vi "WiFiCheck.vi"() -> ()   [LabVIEW 2016]
uses:
  VIs/uPythonX/uPythonX.xctl
panel:
  in  "All Combined":T1(xcontrol)={"VISA Refnum in"="ASRL30::INSTR", "Python Code"="import machine, network, ubinascii, ujson, urequests\nfrom pyb import DAC\nimport utime,math\n\nimport stm\nQSPI = 0xa0001000\nstm.mem32[QSPI] = 0x5000319\nstm.mem32[QSPI+4] = 0x140700\n\nWiFi = network.WLAN()\ndac = DAC(1,buffering=True)            # create DAC 1 on pin X5\n\ndef connect():\n     EN1 = machine.Pin(\"W23\", machine.Pin.OUT, value=1)  # set power high for USB power (500mA now allowed)\n     if not WiFi.isconnected():\n          print (\"Connecting ..\")\n          WiFi.active(True)\n          WiFi.connect(\"Tufts_Wireless\",\"\")\n          i=0\n          while i < 25 and not WiFi.isconnected():\n               utime.sleep_ms(200)\n               i=i+1\n          if WiFi.isconnected():\n               print (\"Connection succeeded\")\n          else:\n               print (\"Connection failed\")     \n\nconnect()\nprint (\"WiFi: \",WiFi.isconnected())\n\n# Info\nTag = \"num\"\nType = \"INT\"\nKey = \"dYy-vDU9TXxDCy2QG3jO4J0s1-QUyYs6sO1xPd1oKQ\"\n\nurlBase = \"https://api.systemlinkcloud.com/nitag/v2/tags/\"\n\nurlValue = urlBase + Tag + \"/values/current\"\n\nheaders = {\"Accept\":\"application/json\",\"x-ni-api-key\":Key}\n\n## GET\n\nwhile True:\n     value = urequests.get(urlValue,headers=headers).text\n     data = ujson.loads(value)\n     result = data.get(\"value\").get(\"value\")\n     print (\"value = \",result)\n     dac.write(int(result))\n     utime.sleep_ms(500)\n     \n     \n"}
  in  "Tell EV3":T1(xcontrol)={"VISA Refnum in"="ASRL30::INSTR", "Python Code"="from pyb import DAC\nimport utime,math\n\ndac = DAC(1,buffering=True)            # create DAC 1 on pin X5\ndac.write(128)          # write a value to the DAC (makes X5 1.65V)\n"}
  in  "SystemLink":T1(xcontrol)={"VISA Refnum in"="ASRL30::INSTR", "Python Code"="import machine, network, ubinascii, ujson, urequests, utime\n\nWiFi = network.WLAN()\n\nmac = ubinascii.hexlify(network.WLAN().config(\"mac\"),\":\").decode()\nprint(\"MAC address: \" + mac)\ndef connect():\n     EN1 = machine.Pin(\"W23\", machine.Pin.OUT, value=1)  # set power high for USB power (500mA now allowed)\n     if not WiFi.isconnected():\n          print (\"Connecting ..\")\n          WiFi.active(True)\n          WiFi.connect(\"Tufts_Wireless\",\"\")\n          i=0\n          while i < 25 and not WiFi.isconnected():\n               utime.sleep_ms(200)\n               i=i+1\n          if WiFi.isconnected():\n               print (\"Connection succeeded\")\n          else:\n               print (\"Connection failed\")     \n\nconnect()\nprint (\"WiFi: \",WiFi.isconnected())\n\n# Info\nTag = \"fred\"\nType = \"STRING\"\nValue = \"hello\"\nKey = \"dYy-vDU9TXxDCy2QG3jO4J0s1-QUyYs6sO1xPd1oKQ\"\n\nurlBase = \"https://api.systemlinkcloud.com/nitag/v2/tags/\"\n     \n## PUT\nurlTag = urlBase + Tag\nurlValue = urlBase + Tag + \"/values/current\"\n\nheaders = {\"Accept\":\"application/json\",\"x-ni-api-key\":Key}\npropName={\"type\":Type,\"path\":Tag}\npropValue = {\"value\":{\"type\":Type,\"value\":Value}}\n\nprint(urequests.put(urlTag,headers=headers,json=propName).text)\nprint(urequests.put(urlValue,headers=headers,json=propValue).text)\n\nurlValue = urlBase + Tag + \"/values/current\"\n\n## GET\nvalue = urequests.get(urlValue,headers=headers).text\n\ndata = ujson.loads(value)\nresult = data.get(\"value\").get(\"value\")\nprint (\"value = \",result)\n"}
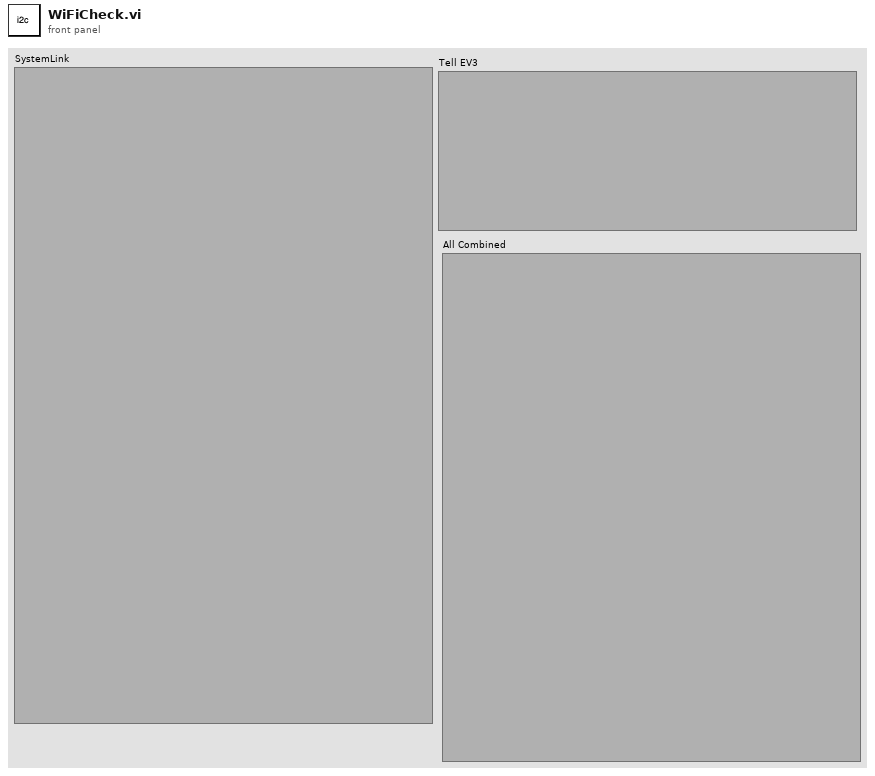
[diagram p1: front panel]
types:
  T1 = cluster{"VISA Refnum in":refnum<visa-resource-name>, "Python Code":string}
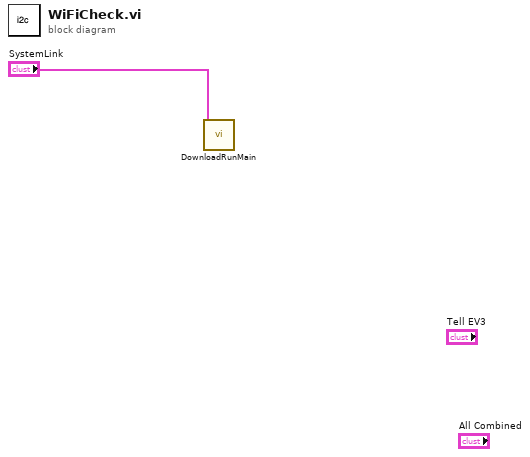
[diagram p0: block diagram]
diagram:
  n1 = call "DownloadRunMain.vi"("Data In"="SystemLink") -> ()  [unwired: 8 in, 3 out]
